vi "QDMH Main 1.vi"(8 "error in (no error)":errorcluster, 10 "Queue Name":string) -> (0 "error out":errorcluster)   [LabVIEW 2013]
doc: "This is a basic Queue Driven Message Handler VI. Most advanced LabVIEW programmers who code extensively in LabVIEW utilitze some variation of this VI. This is a starting point. Some key features need to be added. In particular a robust error handling routine should be added.\n\nAAL 9/09"
uses:
  Users/a0272913/Desktop/2012_AAL Exercises_ Solutions/ExerciseSource/Shared/QDMH Poly VIs/QDMH POLY Enqueue String.vi
panel:
  in  "Launch Dynamic":bool
  out "Message Display":string
  in  "Cancel":bool
  in  "OK":bool
  # "Note:  You must first save the VI and the VI Cluster\nin the same directory as QDMH Main.vit in order for \nthe Launch Dynamic to work."
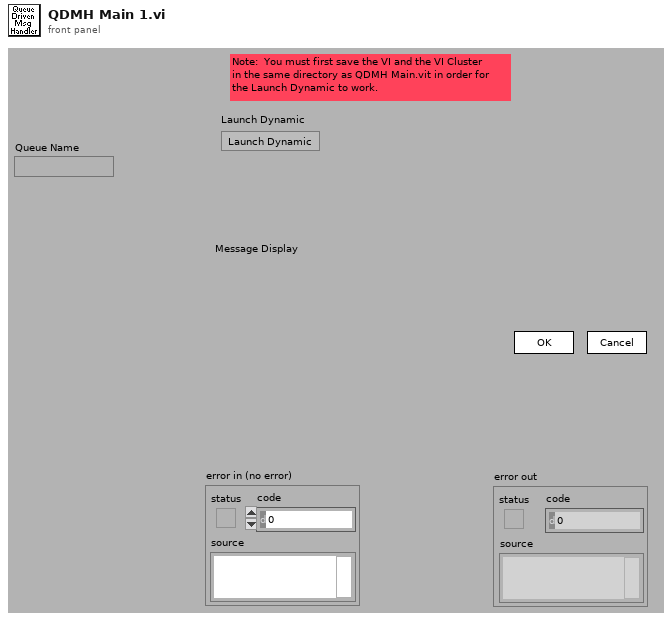
[diagram p1: front panel]
types:
  T1 = cluster{"Operator Name":string, "Current VI's Path":path, "Current VI's  Directory":path, "Queue Names":string[], "# VIs Launched":i32}
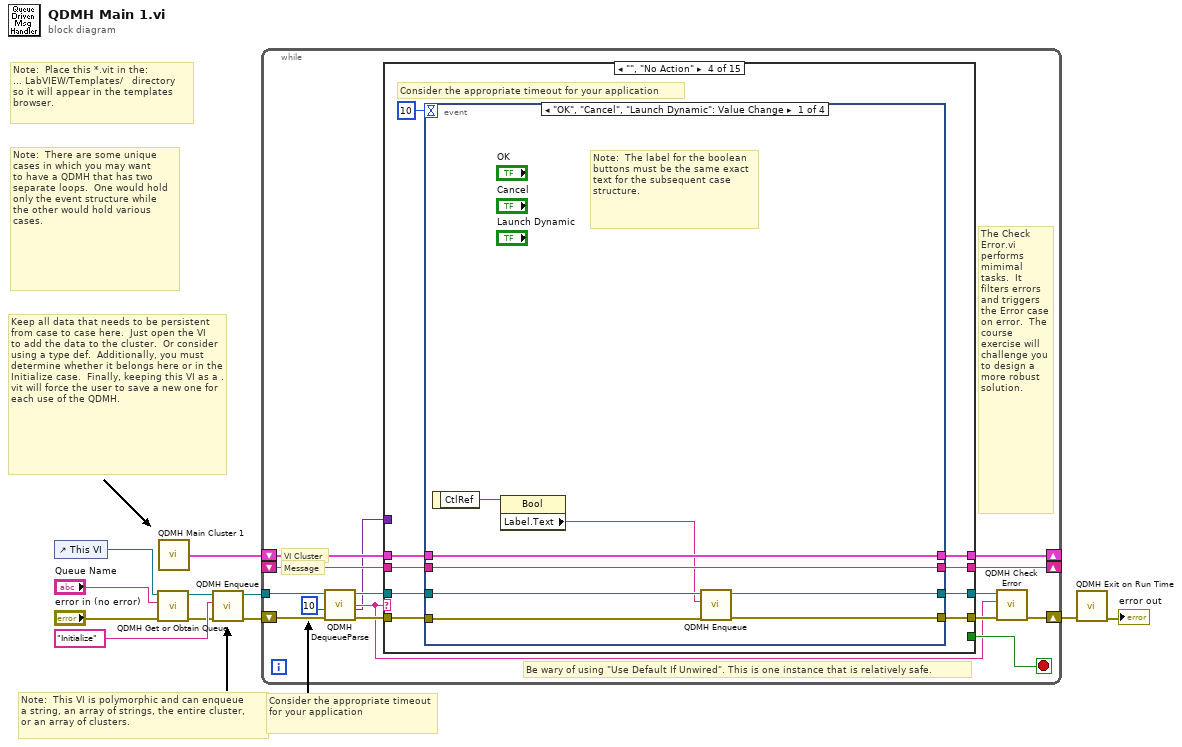
[diagram p0: block diagram]
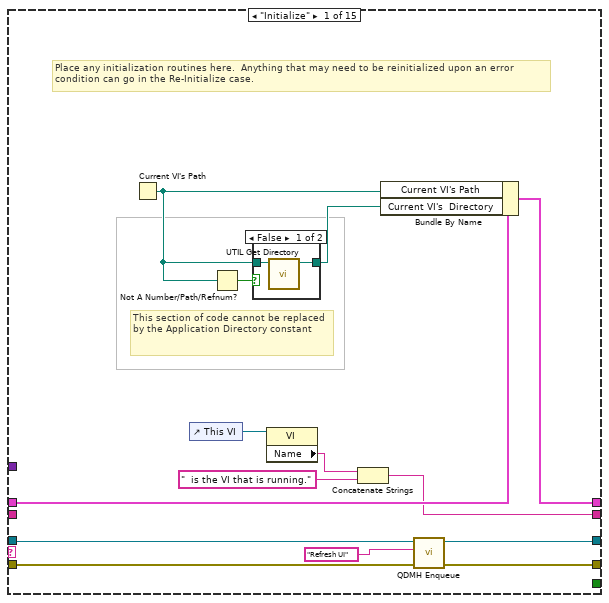
[diagram p2: hidden frame]
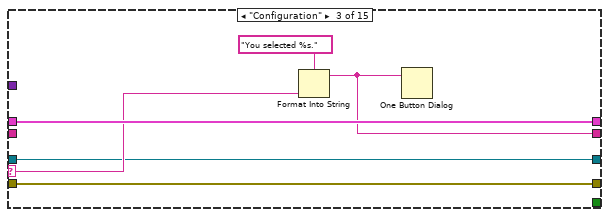
[diagram p5: hidden frame]
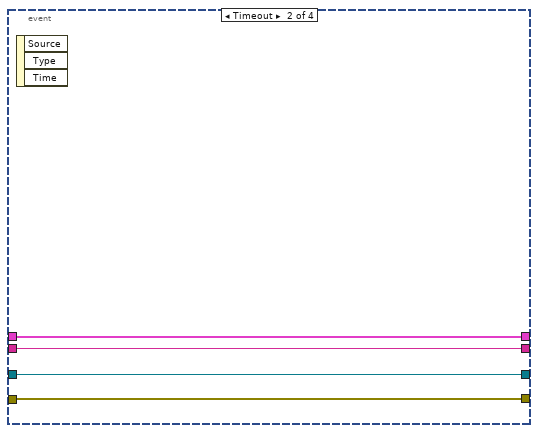
[diagram p6: hidden frame]
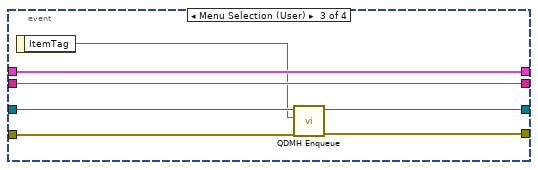
[diagram p7: hidden frame]
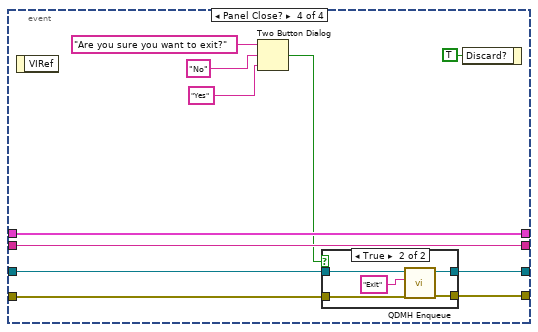
[diagram p8: hidden frame]
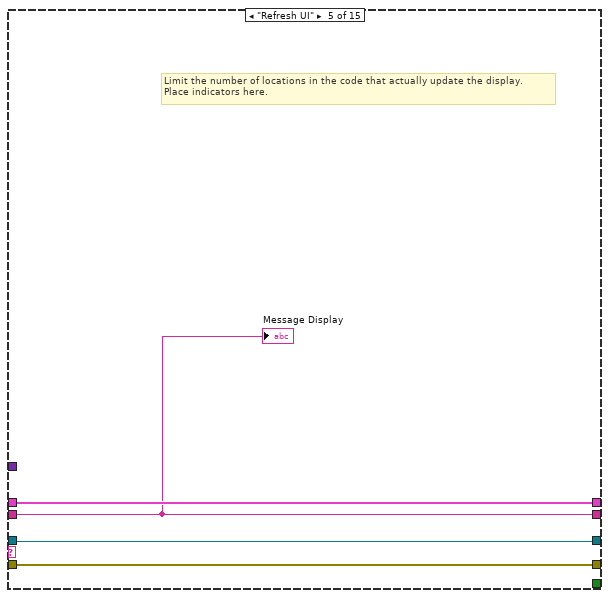
[diagram p10: hidden frame]
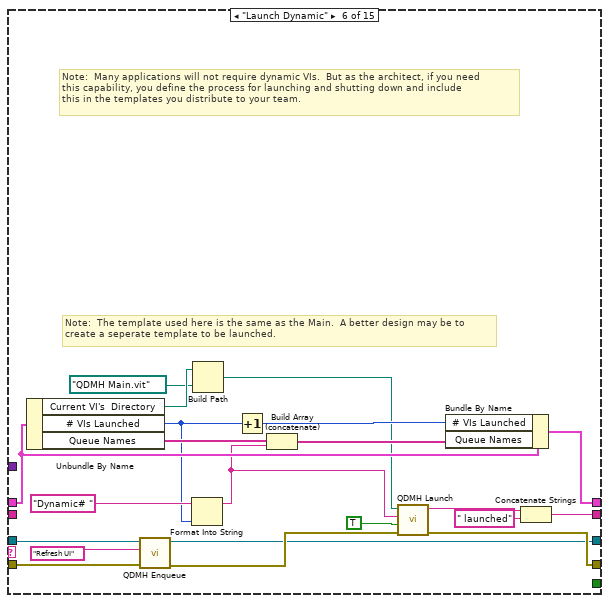
[diagram p11: hidden frame]
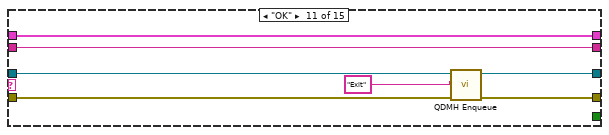
[diagram p16: hidden frame]
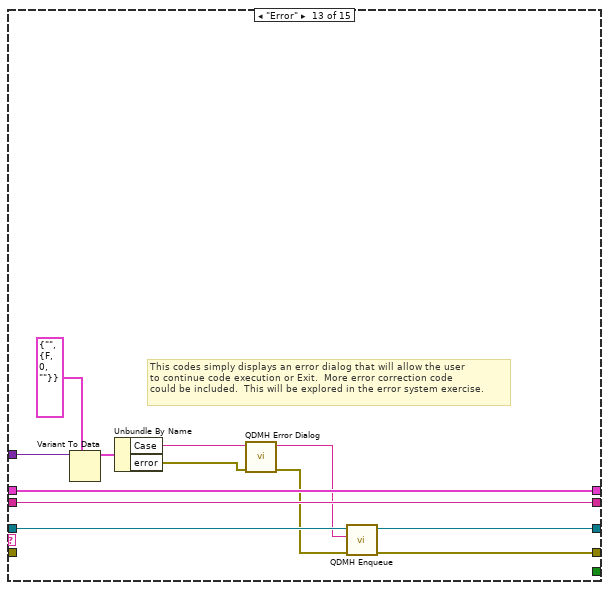
[diagram p18: hidden frame]
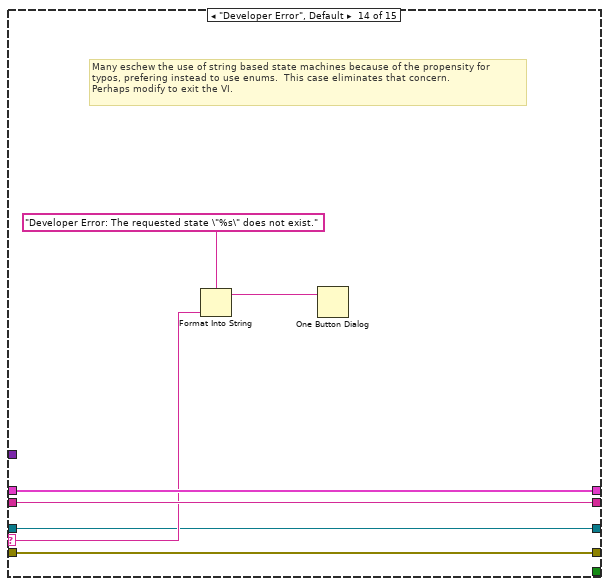
[diagram p19: hidden frame]
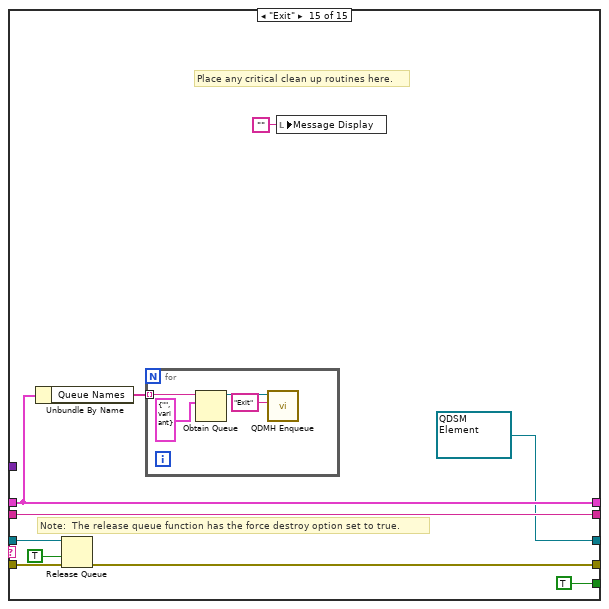
[diagram p20: hidden frame]
diagram:
  # "Consider the appropriate timeout for your application"
  # "Note:  There are some unique\ncases in which you may want\nto have a QDMH that has two\nseparate loops.  One would hold\nonly the event structure while\nthe other would hold various \ncases."
  # "Note:  Place this *.vit in the:\n... LabVIEW/Templates/   directory\nso it will appear in the templates\nbrowser."
  # "Note:  This VI is polymorphic and can enqueue\na string, an array of strings, the entire cluster,\nor an array of clusters."
  # "Keep all data that needs to be persistent\nfrom case to case here.  Just open the VI\nto add the data to the cluster.  Or consider \nusing a type def.  Additionally, you must determine whether it belongs here or in the Initialize case.  Finally, keeping this VI as a .vit will force the user to save a new one for each use of the QDMH."
  n1 = control-ref of="This VI"() -> (w3:refnum<vi>)
  n2 = call "QDMH Get or Obtain Queue.vi"("error in (no error)"="error in (no error)", "Queue Name"="Queue Name", "VI Refnum"=w3) -> ("error out"=w6:errorcluster, "queue out"=w7:refnum<queue>)  [unwired: 7 out]
  n3 = call "QDMH Main Cluster 1.vi"() -> ("Cluster"=w11:T1)
  n4 = call-poly "QDMH Enqueue.vi"("error in (no error)"=w6, "State"="Initialize" ("element"), "queue"=w7) -> ("error out"=w4:errorcluster, "queue out"=w5:refnum<queue>)  [unwired: 7 out]
  n5 = while {
    tunnel: w5 -> [w21]
    shift-left: w11 -> [w22]
    shift-right: [w23] -> _
    shift-left: _ -> [w24]
    shift-right: [w25] -> _
    shift-right: [w15] -> w2
    shift-left: w4 -> [w17]
    stop <- w26 stop-if-true
    # "Be wary of using \"Use Default If Unwired\". This is one instance that is relatively safe."
    # "VI Cluster"
    # "Message"
    # "The Check Error.vi performs mimimal tasks.  It filters errors and triggers the Error case on error.  The course exercise will challenge you to design a more robust solution."
    n6 = call "QDMH DequeueParse.vi"("error in (no error)"=w17, "Timeout"=10 ("ms timeout (-1)"), "queue"=w21) -> ("error out"=w18:errorcluster, "Variant Data"=w12:variant, "State"=w13:string, "queue out"=w19:refnum<queue>)  [unwired: 5 out]
    n7 = case shown="\"\", \"No Action\"" w13 {
      selector: w13 -> [_ _ w50 _ _ _ _ _ _ _ _ _ _ w167 _]
      tunnel: w19 -> [w36 w44 w49 w62 w101 w120 w125 w129 w133 w137 w147 w149 w161 w164 w177]
      tunnel: [_ _ _ _ _ _ _ _ _ _ _ _ _ _ TRUE] -> w26
      tunnel: [w34 w47 w51 w55 w102 w121 w128 w132 w136 w140 w146 w151 w163 w170 w179] -> w25
      tunnel: w24 -> [_ w47 _ w56 w102 _ w128 w132 w136 w140 w146 w151 w163 w170 w179]
      tunnel: [w39 w46 w53 w57 w103 w117 w127 w131 w135 w139 w145 w150 w162 w169 w174] -> w23
      tunnel: w22 -> [w40 w46 w53 w58 w103 w118 w127 w131 w135 w139 w145 w150 w162 w169 w174]
      tunnel: w18 -> [w38 w45 w48 w61 w100 w111 w126 w130 w134 w138 w144 w148 _ w166 w176]
      tunnel: [w37 w45 w48 w60 w100 w110 w126 w130 w134 w138 w143 w148 w160 w166 w171] -> w16
      tunnel: [w29 w44 w49 w54 w101 w107 w125 w129 w133 w137 w141 w149 w159 w164 refnum<queue> refnum ("queue out")] -> w14
      tunnel: w12 -> [_ _ _ _ _ _ _ _ _ _ _ _ w157 _ _]
      frame "Initialize" {
        # "This section of code cannot be replaced by the Application Directory constant"
        # "Place any initialization routines here.  Anything that may need to be reinitialized upon an error\ncondition can go in the Re-Initialize case."
        n8 = Current VI's Path() -> (path=w27:path)
        n9 = control-ref of="This VI"() -> (w33:refnum<vi>)
        n10 = Not A Number/Path/Refnum?(number/path/refnum=w27) -> (NaN/Path/Refnum?=w28:bool)
        n11 = case shown="False" w28 {
          tunnel: w27 -> [w42 w43]
          tunnel: [w41 w43] -> w31
          frame False {
            n12 = call "UTIL Get Directory.vi"("Path In"=w42) -> ("Directory Out"=w41:path)  [unwired: 1 in, 9 out]
          }
          frame True {
          }
        }
        n13 = property class="VI"(reference=w33) -> ("Name"=w32:string)  [unwired: 1 in, 2 out]
        n14 = Concatenate Strings(w32, "  is the VI that is running." ("string")) -> (w34:string)
        n15 = Bundle By Name(cluster=w40, "Current VI's Path"=w27, "Current VI's  Directory"=w31) -> (w39:T1)
        n16 = call-poly "QDMH Enqueue.vi"("error in (no error)"=w38, "State"="Refresh UI" ("New State"), "queue"=w36) -> ("error out"=w37:errorcluster, "queue out"=w29:refnum<queue>)  [unwired: 7 out]
      }
      frame "Re-Initialize" {
        # "This case includes initialization functionality that may need to run again during the course of the VI"
      }
      frame "Configuration" {
        n17 = Format Into String(format string="You selected %s." ("Format String"), w50) -> (resulting string=w51:string)  [unwired: 2 in, 1 out]
        n18 = One Button Dialog(message=w51) -> ()  [unwired: 2 out]
      }
      frame "", "No Action" {
        # "Consider the appropriate timeout for your application"
        n19 = event shown="[0] \"OK\", \"Cancel\", \"Launch Dynamic\": Value Change" {
          selector: _ -> [_ _ _ _]
          dyn-events: _ -> [_ _ _ _]
          timeout: 10 -> [_ _ _ _]
          tunnel: w62 -> [w69 w71 w81 w87]
          tunnel: [w68 w74 w79 w84] -> w60
          tunnel: w61 -> [w67 w74 w80 w85]
          tunnel: w58 -> [w66 w73 w78 w92]
          tunnel: [w66 w73 w78 w92] -> w57
          tunnel: w56 -> [w65 w72 w77 w91]
          tunnel: [w65 w72 w77 w91] -> w55
          tunnel: [w63 w71 w75 w86] -> w54
          event "OK", "Cancel", "Launch Dynamic": Value Change {
            # "Note:  The label for the boolean buttons must be the same exact text for the subsequent case structure."
            n20 = event-data() -> ("CtlRef"=w70:refnum<vi>)  [unwired: 1 out]
            n21 = property class="Bool"(reference=w70) -> ("Label.Text"=w64:string)  [unwired: 1 in, 2 out]
            n22 = call-poly "QDMH Enqueue.vi"("error in (no error)"=w67, "State"=w64, "queue"=w69) -> ("error out"=w68:errorcluster, "queue out"=w63:refnum<queue>)  [unwired: 7 out]
          }
          event Timeout {
            n23 = event-data() -> ()  [unwired: 4 out]
          }
          event Menu Selection (User) {
            n24 = event-data() -> ("ItemTag"=w76:string)  [unwired: 1 out]
            n25 = call-poly "QDMH Enqueue.vi"("error in (no error)"=w80, "State"=w76, "queue"=w81) -> ("error out"=w79:errorcluster, "queue out"=w75:refnum<queue>)  [unwired: 7 out]
          }
          event Panel Close? {
            n26 = event-data() -> ()  [unwired: 2 out]
            n27 = Two Button Dialog(message="Are you sure you want to exit?", 1:"Yes" ("F button name (\"Cancel\")"), 2:"No" ("T button name (\"OK\")")) -> (T button?=w83:bool)
            n28 = case shown="True" w83 {
              tunnel: w87 -> [w94 w99]
              tunnel: [w94 w98] -> w86
              tunnel: w85 -> [w93 w97]
              tunnel: [w93 w96] -> w84
              frame False {
              }
              frame True {
                n29 = call-poly "QDMH Enqueue.vi"("error in (no error)"=w97, "State"="Exit", "queue"=w99) -> ("error out"=w96:errorcluster, "queue out"=w98:refnum<queue>)  [unwired: 7 out]
              }
            }
            n30 = event-data("Discard?"=TRUE) -> ()  [unwired: 1 in, 1 out]
          }
        }
      }
      frame "Refresh UI" {
        # "Limit the number of locations in the code that actually update the display.\nPlace indicators here."
        "Message Display" <- w102
      }
      frame "Launch Dynamic" {
        # "Note:  The template used here is the same as the Main.  A better design may be to\ncreate a seperate template to be launched."
        # "Note:  Many applications will not require dynamic VIs.  But as the architect, if you need\nthis capability, you define the process for launching and shutting down and include\nthis in the templates you distribute to your team."
        n31 = Unbundle By Name(w118) -> ("Current VI's  Directory"=w106:path, "# VIs Launched"=w114:i32, "Queue Names"=w116:string[])
        n32 = call-poly "QDMH Enqueue.vi"("error in (no error)"=w111, "State"="Refresh UI" ("New State"), "queue"=w120) -> ("error out"=w109:errorcluster, "queue out"=w107:refnum<queue>)  [unwired: 7 out]
        n33 = Format Into String(initial string="Dynamic# ", w114) -> (resulting string=w112:string)  [unwired: 2 in, 1 out]
        n34 = Build Path(base path=w106, name or relative path=path "QDMH Main.vit" ("vi path")) -> (appended path=w104:path)
        n35 = Increment(x=w114) -> (x+1=w113:i32)
        n36 = Build Array (concatenate)(w116, w112) -> (w115:string[])
        n37 = call "QDMH Launch.vi"("error in (no error)"=w109, "Front Panel Window (Open)"=TRUE ("Front Panel Window:Open"), "Queue Name"=w112, "VI Path"=w104) -> ("error out"=w110:errorcluster, "Launched VI Name"=w123:string)  [unwired: 6 out]
        n38 = Bundle By Name(cluster=w118, "# VIs Launched"=w113, "Queue Names"=w115) -> (w117:T1)
        n39 = Concatenate Strings(w123, " launched" ("string")) -> (w121:string)
      }
      frame "Shutdown Dynamic" {
      }
      frame "Send Message to Dynamic" {
      }
      frame "Receive Message From Dynamic" {
      }
      frame "<duplicate me for new states >" {
        # "Duplicate this state for any additional states that you add."
      }
      frame "OK" {
        n40 = call-poly "QDMH Enqueue.vi"("error in (no error)"=w144, "State"="Exit" ("New State"), "queue"=w147) -> ("error out"=w143:errorcluster, "queue out"=w141:refnum<queue>)  [unwired: 7 out]
      }
      frame "Cancel" {
      }
      frame "Error" {
        # "This codes simply displays an error dialog that will allow the user\nto continue code execution or Exit.  More error correction code\ncould be included.  This will be explored in the error system exercise."
        n41 = Variant To Data(type=cluster{"Case":string, "error":errorcluster} {"Case"="", "error"={"status"=FALSE, "code"=0, "source"=""}} ("QDSM Element"), Variant=w157) -> (data=w156:cluster{"Case":string, "error":errorcluster})  [unwired: 1 in, 1 out]
        n42 = Unbundle By Name(w156) -> ("Case"=w155:string, "error"=w154:errorcluster)
        n43 = call "QDMH Error Dialog.vi"("error"=w154, "Case Error Occured"=w155) -> ("error out (no error)"=w152:errorcluster, "Case to Execute"=w153:string)  [unwired: 8 out]
        n44 = call-poly "QDMH Enqueue.vi"("error in (no error)"=w152, "State"=w153, "queue"=w161) -> ("error out"=w160:errorcluster, "queue out"=w159:refnum<queue>)  [unwired: 7 out]
      }
      frame "Developer Error", Default {
        # "Many eschew the use of string based state machines because of the propensity for\ntypos, prefering instead to use enums.  This case eliminates that concern.\nPerhaps modify to exit the VI."
        n45 = Format Into String(format string="Developer Error: The requested state \"%s\" does not exist." ("message"), w167) -> (resulting string=w165:string)  [unwired: 2 in, 1 out]
        n46 = One Button Dialog(message=w165) -> ()  [unwired: 2 out]
      }
      frame "Exit" {
        # "Note:  The release queue function has the force destroy option set to true."
        # "Place any critical clean up routines here."
        n47 = Unbundle By Name(w174) -> ("Queue Names"=w172:string[])
        n48 = Release Queue(queue=w177, force destroy? (F)=TRUE, error in (no error)=w176) -> (error out=w171:errorcluster)  [unwired: 2 out]
        n49 = for {
          tunnel: w172 -> [w184] mode=indexing
          n50 = Obtain Queue(name (unnamed)=w184, element data type=cluster{"State":string, "Variant Data":variant} {"State"="", "Variant Data"=variant} ("QDSM Element")) -> (queue out=w183:refnum<queue>)  [unwired: 3 in, 2 out]
          n51 = call-poly "QDMH Enqueue.vi"("State"="Exit" ("element"), "queue"=w183) -> ()  [unwired: 1 in, 9 out]
        }
        n52 = local write "Message Display"("") -> ()
      }
    }
    n53 = call "QDMH Check Error.vi"("error in (no error)"=w16, "Case"=w13, "queue"=w14) -> ("error out"=w15:errorcluster)  [unwired: 1 in, 7 out]
  }
  n54 = call "QDMH Exit on Run Time.vi"("error in (no error)"=w2) -> ("error out"=→"error out":errorcluster)  [unwired: 10 in]
